vi "On Device Selected (SubVI).vi"(0 "CmdLib In":refnum<k24>, 5 "Device Key":string, 7 "Device Key In":string, 9 "Device Array":T1(array[cluster]), 11 "error in":errorcluster) -> (6 "Device Address":i32, 10 "Device Key Out":string, 15 "error out":errorcluster)   [LabVIEW 2017]
doc: "by Tanguy BOULARD"
uses:
  dll/CmdLib.dll
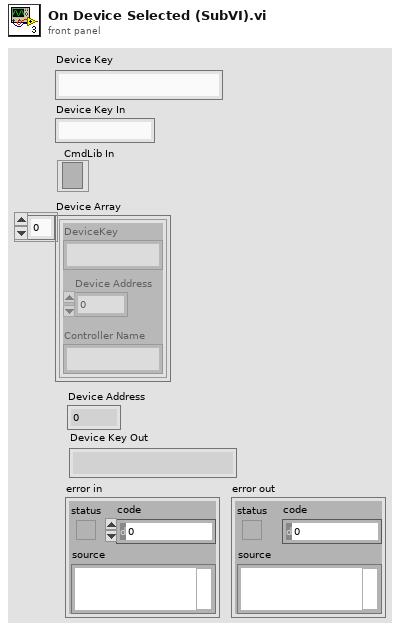
[diagram p1: front panel]
types:
  T1 = cluster{"DeviceKey":string, "Device Address":i32, "Controller Name":string}[]
  T2 = cluster{"DeviceKey":string, "Device Address":i32, "Controller Name":string}
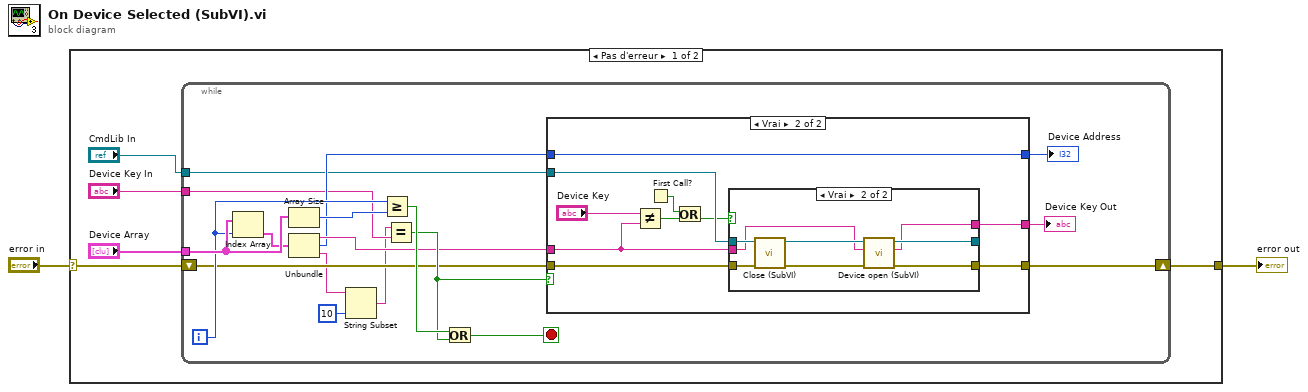
[diagram p0: block diagram]
diagram:
  n1 = case shown="Pas d'erreur" "error in" {
    selector: "error in" -> [w4 w50]
    tunnel: [w6 w50] -> w2
    frame No Error {
      n2 = while {
        tunnel: "Device Array" -> [w24]
        tunnel: "Device Key In" -> [w13]
        shift-right: [w16] -> w6
        shift-left: w4 -> [w15]
        tunnel: "CmdLib In" -> [w14]
        i -> [w23]
        stop <- w19 stop-if-true
        n3 = Index Array(array=w24, index=w23) -> (element=w22:T2)
        n4 = Array Size(array=w24) -> (size(s)=w25:i32)
        n5 = Unbundle(w22) -> ("DeviceKey"=w18:string, "Device Address"=w17:i32, "Controller Name"=w11:string)
        n6 = String Subset(string=w11, length (rest)=10 ("longueur (reste)")) -> (substring=w12:string)  [unwired: 1 in]
        n7 = Greater Or Equal?(x=w23, y=w25) -> (x >= y?=w21:bool)
        n8 = Equal?(x=w12, y=w13) -> (x = y?=w20:bool)
        n9 = Or(x=w21, y=w20) -> (x .or. y?=w19:bool)
        n10 = case shown="Vrai" w20 {
          tunnel: w18 -> [w27 w37]
          tunnel: w17 -> [w26 w29]
          tunnel: [w28 w33] -> w16
          tunnel: w15 -> [w28 w38]
          tunnel: w14 -> [_ w35]
          tunnel: [w27 w30] -> w9
          tunnel: [w26 w29] -> w8
          frame False {
          }
          frame True {
            n11 = Not Equal?(x="Device Key", y=w37) -> (x != y?=w36:bool)
            n12 = First Call?() -> (First Call?: T/F=w31:bool)
            n13 = Or(x=w31, y=w36) -> (x .or. y?=w32:bool)
            n14 = case shown="Vrai" w32 {
              tunnel: [w41 w44] -> w33
              tunnel: w35 -> [w40 w49]
              tunnel: w38 -> [w41 w47]
              tunnel: w37 -> [w39 w45]
              tunnel: [w40 w43] -> _
              tunnel: [w39 w42] -> w30
              frame False {
              }
              frame True {
                n15 = call "Close (SubVI).vi"("error in"=w47, "CmdLib In"=w49) -> ("error out"=w48:errorcluster, "CmdLib Out"=w46:refnum<k24>)  [unwired: 8 in]
                n16 = call "Device open (SubVI).vi"("error in (no error)"=w48, "DeviceKey In"=w45, "CmdLib In"=w46) -> ("error out"=w44:errorcluster, "DeviceKey Out"=w42:string, "CmdLib Out"=w43:refnum<k24>)  [unwired: 6 in]
              }
            }
          }
        }
        "Device Key Out" <- w9
        "Device Address" <- w8
      }
    }
    frame Error {
    }
  }
  "error out" <- w2
